vi "test.network.ipReporter.vi"() -> ()   [LabVIEW 2017]
uses:
  Network/IP Reporter/_Typedef/Def-IniSettings -- Cluster.ctl
  8ed771ae-4439-4f02-8ca7-f9c939418156.vi
panel:
  in  "notification":string
  in  "stop":bool
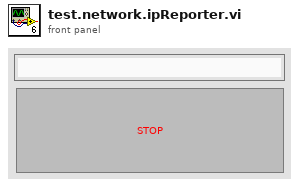
[diagram p1: front panel]
types:
  T1 = typedef "Def-IniSettings -- Cluster.ctl" = cluster{"address":string, "receiver port":u16, "Ignore Gateway IP":bool, "HostName":string}
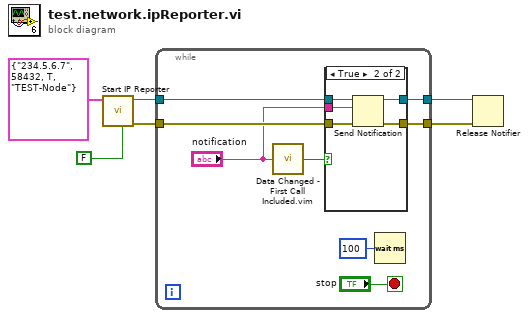
[diagram p0: block diagram]
diagram:
  n1 = call "Start IP Reporter.vi"("ignore Gateway IP?(T)"=FALSE ("Load From File(F)"), "Setttings"=T1 {"address"="234.5.6.7", "receiver port"=58432, "Ignore Gateway IP"=TRUE, "HostName"="TEST-Node"}) -> ("error out"=w5:errorcluster, "Information Notifier"=w4:refnum<notifier>)  [unwired: 8 in]
  n2 = while {
    tunnel: w5 -> [w11]
    tunnel: w4 -> [w12]
    tunnel: [w10] -> w3
    tunnel: [w9] -> w2
    stop <- "stop" stop-if-true
    n3 = call "Data Changed - First Call Included.vim"("Variant"="notification") -> ("Changed"=w7:bool)
    n4 = case shown="True" w7 {
      tunnel: w12 -> [w16 w21]
      tunnel: w11 -> [w15 w20]
      tunnel: [w16 w19] -> w10
      tunnel: [w15 w18] -> w9
      tunnel: "notification" -> [_ w17]
      frame False {
      }
      frame True {
        n5 = Send Notification(notification=w17, notifier=w21, error in (no error)=w20) -> (notifier out=w19:refnum<notifier>, error out=w18:errorcluster)
      }
    }
    n6 = Wait (ms)(milliseconds to wait=u32 100) -> ()  [unwired: 1 out]
  }
  n7 = Release Notifier(notifier=w3, error in (no error)=w2) -> ()  [unwired: 1 in, 3 out]
